vi "Read Bitmap.vi"(8 "error in (no error)":errorcluster, 11 "Bitmap Canvas in":refnum<class "Bitmap Canvas.lvclass">) -> (0 "error out":errorcluster, 2 "Bitmap":u32[][](array[numeric]), 3 "Bitmap Canvas out":refnum<class "Bitmap Canvas.lvclass">)   [LabVIEW 2023, in "Font Glyph Drawer Interface.lvlib" / "Bitmap Canvas.lvclass"]
uses:
  Bitmap Canvas.lvclass
  Bitmap Canvas.lvclass/Bitmap Canvas.ctl
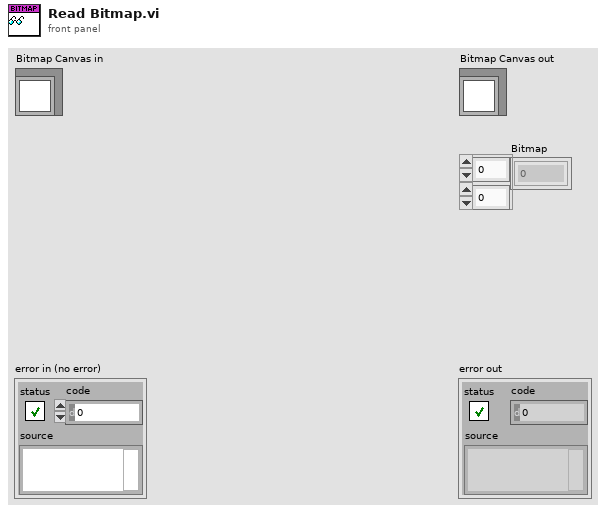
[diagram p1: front panel]
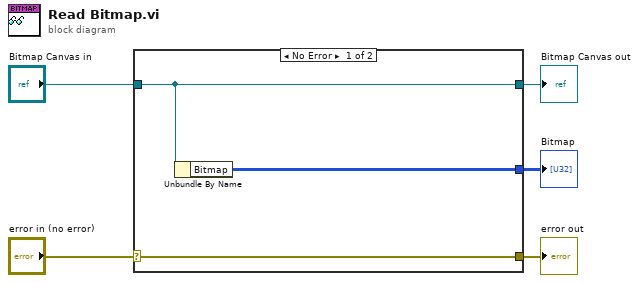
[diagram p0: block diagram]
diagram:
  n1 = case shown="No Error" "error in (no error)" {
    selector: "error in (no error)" -> [w8 w9]
    tunnel: [w8 w9] -> w4
    tunnel: [w7 w10] -> w2
    tunnel: "Bitmap Canvas in" -> [w7 w10]
    tunnel: [w6 _] -> w1
    frame No Error {
      n2 = Unbundle By Name(w7) -> ("Bitmap"=w6:u32[][])
    }
    frame Error {
    }
  }
  "error out" <- w4
  "Bitmap Canvas out" <- w2
  "Bitmap" <- w1
